vi "Get FPGA Reference.vi"(0 "session in":refnum<class "Digitizer Control.lvclass">, 5 "error in (no error)":errorcluster) -> (14 "session out":refnum<class "Digitizer Control.lvclass">, 15 "fpga reference":refnum<k20>, 19 "error out":errorcluster)   [LabVIEW 2021, in "Digitizer Control.lvclass"]
doc: "Returns the FPGA Target reference.\n\nInput:\n\n<B>session in</B>: The device session.\n\nOutputs:\n\n<B>session out</B>: The device session passed on the <B>session in</B> input.\n\n<B>fpga reference</B>: The FPGA Target reference."
uses:
  Digitizer Control.lvclass
  Digitizer Control.lvclass/Digitizer Control.ctl
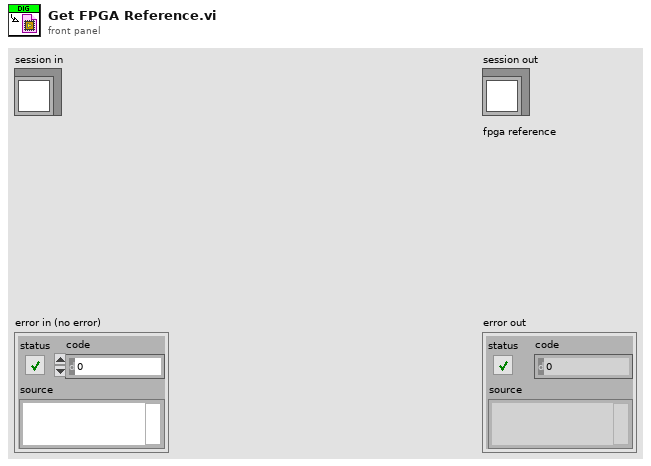
[diagram p1: front panel]
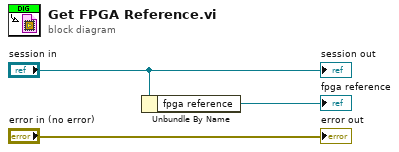
[diagram p0: block diagram]
diagram:
  n1 = Unbundle By Name("session in") -> ("fpga reference"=→"fpga reference":refnum<k20>)
  "error out" <- "error in (no error)"
  "session out" <- "session in"
